vi "Destroy.vi"(0 "reference in":refnum<class "Subject Controller.lvclass">, 5 "error in (no error)":errorcluster) -> (14 "reference out":refnum<class "Subject Controller.lvclass">, 19 "error out":errorcluster)   [LabVIEW 2015, in "Subject Controller.lvclass"]
doc: "Destructor."
uses:
  Subject Controller.lvclass
  <vilib>/addons/_AddQ/G#Object/G#Object.lvclass
  APP/subject_class/subject.lvclass
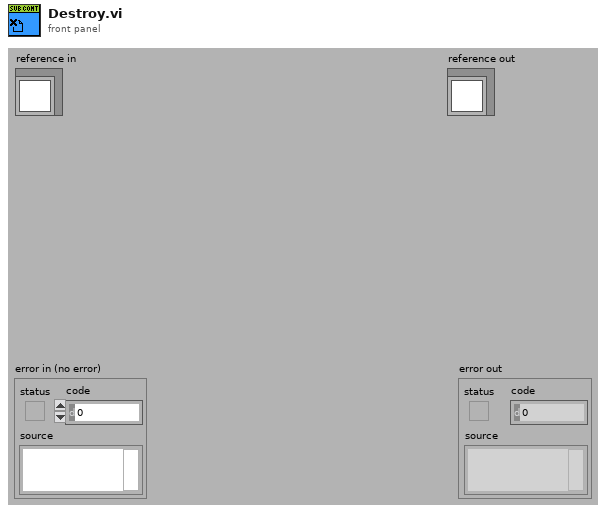
[diagram p1: front panel]
types:
  T1 = typedef "Subject Controller.lvclass/ObjectAttributes.ctl" = cluster{"MyAttribute":dbl, "subject_controller_ref":refnum<class "Subject Controller.lvclass">, "file_controller_ref":refnum<class "File Controller.lvclass">, "subject_refs":refnum<class "subject.lvclass">[], "subjectIndex":i32, "file_type":T2}
  T2 = typedef "excelFile.lvclass/fileType.ctl" = enum16{"database", "CosmedTest"}
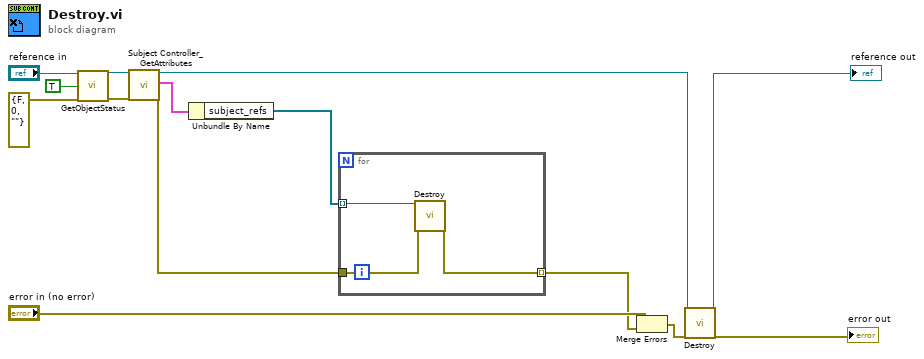
[diagram p0: block diagram]
diagram:
  n1 = call-dynamic "GetObjectStatus.vi"("reference in"="reference in", "simple info (F)"=TRUE ("simple info"), "error in (no error)"=errorcluster {"status"=FALSE, "code"=0, "source"=""}) -> ("reference out"=w8:refnum<class "Subject Controller.lvclass">, "error out"=w9:errorcluster)  [unwired: 5 in, 10 out]
  n2 = call "Subject Controller_GetAttributes.vi"("reference in"=w8, "error in (no error)"=w9) -> ("reference out"=w7:refnum<class "Subject Controller.lvclass">, "attributes"=w6:T1, "error out"=w2:errorcluster)  [unwired: 14 in, 1 out]
  n3 = Unbundle By Name(w6) -> ("subject_refs"=w3:refnum<class "subject.lvclass">[])
  n4 = for {
    tunnel: w3 -> [w17] mode=indexing
    tunnel: w2 -> [w16]
    tunnel: [w15] -> w1 mode=indexing
    n5 = call-dynamic "Destroy.vi"("reference in"=w17, "error in (no error)"=w16) -> ("error out"=w15:errorcluster)  [unwired: 16 in, 1 out]
  }
  n6 = Merge Errors("error in (no error)", w1) -> (w13:errorcluster)
  n7 = call-parent "Destroy.vi"("reference in"=w7, "error in (no error)"=w13) -> ("reference out"=→"reference out":refnum<class "Subject Controller.lvclass">, "error out"=→"error out":errorcluster)  [unwired: 16 in]
